vi "DistanceBetween.vi"(1 "B":T1, 2 "A":T1) -> (0 "Dist(A,B)":dbl format="%#_13g")   [LabVIEW 2017, in "Atom.lvclass"]
uses:
  Atom.lvclass
  Common/Position.ctl
  Common/Common.lvlib
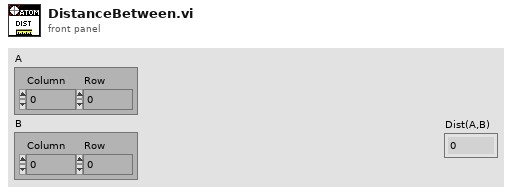
[diagram p1: front panel]
types:
  T1 = typedef "Common.lvlib/Position.ctl" = cluster{"Column":i32, "Row":i32}
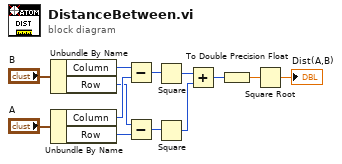
[diagram p0: block diagram]
diagram:
  n1 = Unbundle By Name("B") -> ("Column"=w11:i32, "Row"=w8:i32)
  n2 = Unbundle By Name("A") -> ("Column"=w10:i32, "Row"=w7:i32)
  n3 = Subtract(x=w11, y=w10) -> (x-y=w9:i32)
  n4 = Subtract(x=w8, y=w7) -> (x-y=w6:i32)
  n5 = Square(x=w9) -> (x^2=w2:i32)
  n6 = Square(x=w6) -> (x^2=w3:i32)
  n7 = Add(x=w2, y=w3) -> (x+y=w1:i32)
  n8 = To Double Precision Float(number=w1) -> (double precision float=w5:dbl)
  n9 = Square Root(x=w5) -> (sqrt(x)=→"Dist(A,B)":dbl)
